vi "registers to data.vi"(6 "word order":T1, 9 "specifications":T2[](array[typedef]), 10 "registers":u16[](array[numeric]), 11 "allocation":T4) -> (3 "data table":T4)   [LabVIEW 2015, in "Modbus Module runtime.lvclass"]
uses:
  Modbus Module runtime.lvclass
  <vilib>/NI/Tag Bus/table/data table.ctl
  data mapping elements.ctl
  <vilib>/NI/Tag Bus/tag/Data Type.ctl
  <vilib>/NI/Tag Bus/table/data polymorphs/write one/write Double.vi
  <vilib>/NI/Tag Bus/table/data polymorphs/write one/write Single.vi
  <vilib>/NI/Tag Bus/table/data polymorphs/write one/write I64.vi
  <vilib>/NI/Tag Bus/table/data polymorphs/write one/write U64.vi
  <vilib>/NI/Tag Bus/table/data polymorphs/write one/write I32.vi
  <vilib>/NI/Tag Bus/table/data polymorphs/write one/write U32.vi
  <vilib>/NI/Tag Bus/table/data polymorphs/write one/write I16.vi
  <vilib>/NI/Tag Bus/table/data polymorphs/write one/write U16.vi
  <vilib>/NI/Tag Bus/table/data polymorphs/write one/write I8.vi
  <vilib>/NI/Tag Bus/table/data polymorphs/write one/write U8.vi
  <vilib>/NI/Tag Bus/table/data polymorphs/write one/write String.vi
  <vilib>/NI/Tag Bus/table/data polymorphs/write one/write Boolean.vi
  <vilib>/NI/Tag Bus/table/data table.lvlib
  <vilib>/NI/Tag Bus/tag/tag descriptor.lvclass
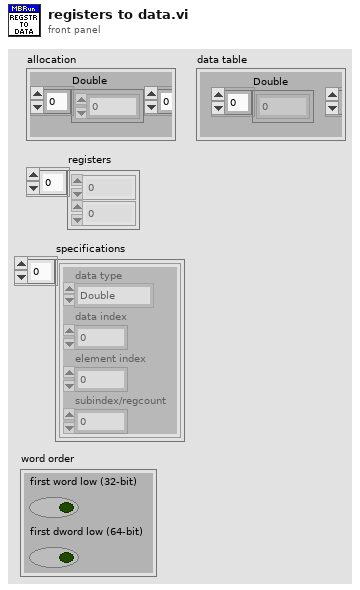
[diagram p1: front panel]
types:
  T1 = cluster{"first word low (32-bit)":bool, "first dword low (64-bit)":bool}
  T2 = typedef "Modbus Module runtime.lvclass/data mapping elements.ctl" = cluster{"data type":T3, "data index":i32, "element index":i32, "subindex/regcount":i32}
  T3 = typedef "tag bus.lvlib/tag descriptor.lvclass/Data Type.ctl" = enum16{"Double", "Single", "I64", "I32", "I16", "I8", "U64", "U32", "U16", "U8", "Boolean", "String", "Array of Double", "Array of Single", "Array of I64", "Array of I32", "Array of I16", "Array of I8", "Array of U64", "Array of U32", "Array of U16", "Array of U8", "Array of Boolean", "Array of String"}
  T4 = typedef "tag bus.lvlib/data table.lvlib/data table.ctl" = cluster{"Double":dbl[], "Single":sgl[], "I64":i64[], "I32":i32[], "I16":i16[], "I8":i8[], "U64":u64[], "U32":u32[], "U16":u16[], "U8":u8[], "Boolean":bool[], "String":string[], "Array of Double":cluster{"DBL Array":dbl[]}[], "Array of Single":cluster{"SGL Array":sgl[]}[], "Array of I64":cluster{"I64 Array":i64[]}[], "Array of I32":cluster{"I32 Array":i32[]}[], "Array of I16":cluster{"I16 Array":i16[]}[], "Array of I8":cluster{"I8 Array":i8[]}[], "Array of U64":cluster{"U64 Array":u64[]}[], "Array of U32":cluster{"U32 Array":u32[]}[], "Array of U16":cluster{"U16 Array":u16[]}[], "Array of U8":cluster{"U8 Array":u8[]}[], "Array of Boolean":cluster{"Boolean Array":bool[]}[], "Array of String":cluster{"String Array":string[]}[]}
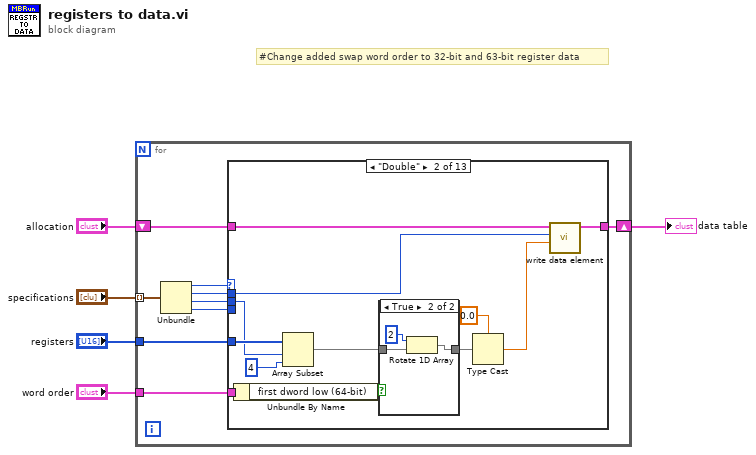
[diagram p0: block diagram]
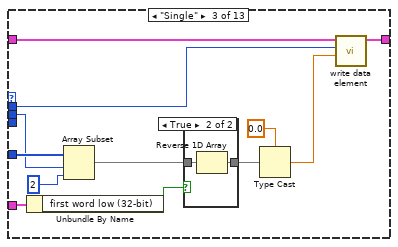
[diagram p4: hidden frame]
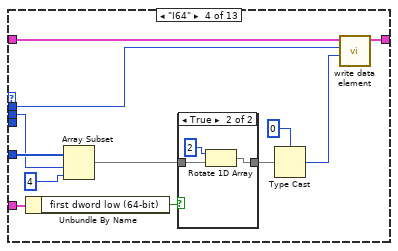
[diagram p6: hidden frame]
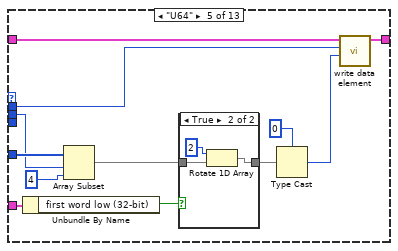
[diagram p8: hidden frame]
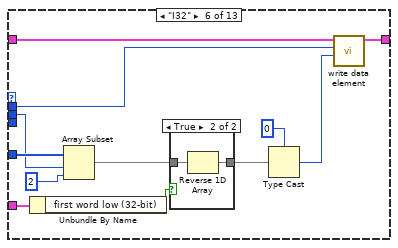
[diagram p10: hidden frame]
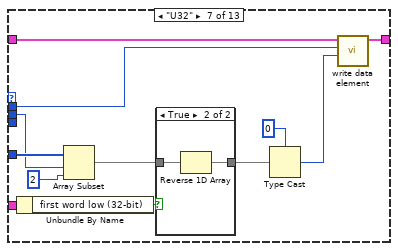
[diagram p12: hidden frame]
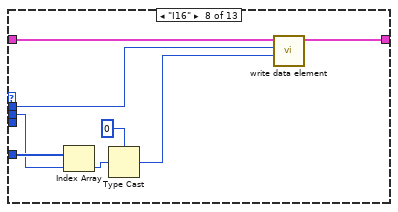
[diagram p14: hidden frame]
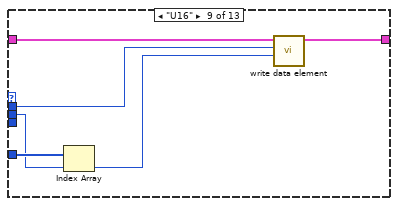
[diagram p15: hidden frame]
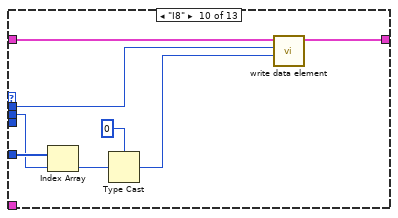
[diagram p16: hidden frame]
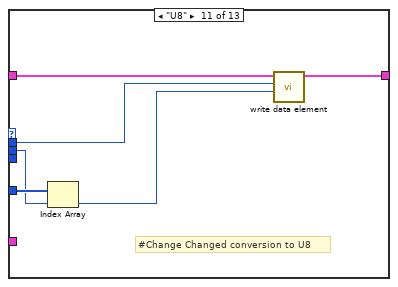
[diagram p17: hidden frame]
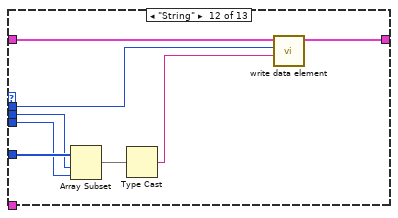
[diagram p18: hidden frame]
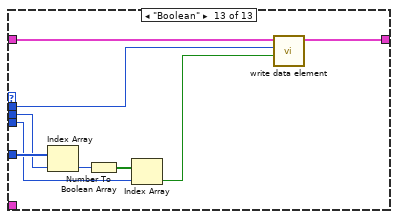
[diagram p19: hidden frame]
diagram:
  # "#Change added swap word order to 32-bit and 63-bit register data"
  n1 = for {
    shift-right: [w11] -> w4
    shift-left: "allocation" -> [w12]
    tunnel: "registers" -> [w10]
    tunnel: "specifications" -> [w14] mode=indexing
    tunnel: "word order" -> [w6]
    n2 = Unbundle(w14) -> ("data type"=w13:T3, "data index"=w9:i32, "element index"=w7:i32, "subindex/regcount"=w8:i32)
    n3 = case shown="\"Double\"" w13 {
      tunnel: w12 -> [w15 w27 w43 w58 w74 w90 w105 w116 w122 w130 w136 w144 w153]
      tunnel: [w15 w26 w42 w57 w73 w89 w104 w115 w121 w129 w135 w143 w152] -> w11
      tunnel: w7 -> [_ w23 w39 w54 w70 w86 w101 w113 w119 w127 w133 w140 w150]
      tunnel: w10 -> [_ w25 w41 w56 w72 w88 w103 w114 w120 w128 w134 w141 w151]
      tunnel: w9 -> [_ w22 w38 w53 w69 w85 w100 w112 w118 w126 w132 w142 w149]
      tunnel: w8 -> [_ _ _ _ _ _ _ _ _ _ _ w139 w145]
      tunnel: w6 -> [_ w19 w35 w48 w66 w82 w97 _ _ _ _ _ _]
      frame Default {
      }
      frame "Double" {
        n4 = Unbundle By Name(w19) -> ("first dword low (64-bit)"=w18:bool)
        n5 = Array Subset(array=w25, index=w23, length=4 ("x")) -> (w17:u16[])
        n6 = case shown="True" w18 {
          tunnel: w17 -> [w28 w31]
          tunnel: [w28 w29] -> w16
          frame False {
          }
          frame True {
            n7 = Rotate 1D Array(1:w31, 2:2 ("n")) -> (0:w29:u16[])
          }
        }
        n8 = Type Cast(type=0.0, x=w16) -> (*(type *) &x=w20:dbl)
        n9 = call-poly <vilib>:"write data element.vi"("value"=w20, "index"=w22, "data table in"=w27) -> ("data table out"=w26:T4)  [unwired: 8 in]
      }
      frame "Single" {
        n10 = Unbundle By Name(w35) -> ("first word low (32-bit)"=w34:bool)
        n11 = Array Subset(array=w41, index=w39, length=2 ("x")) -> (w33:u16[])
        n12 = case shown="True" w34 {
          tunnel: w33 -> [w44 w46]
          tunnel: [w44 w45] -> w32
          frame False {
          }
          frame True {
            n13 = Reverse 1D Array(array=w46) -> (reversed array=w45:u16[])
          }
        }
        n14 = Type Cast(type=sgl 0.0, x=w32) -> (*(type *) &x=w36:sgl)
        n15 = call-poly <vilib>:"write data element.vi"("value"=w36, "index"=w38, "data table in"=w43) -> ("data table out"=w42:T4)  [unwired: 8 in]
      }
      frame "I64" {
        n16 = Unbundle By Name(w48) -> ("first dword low (64-bit)"=w47:bool)
        n17 = Array Subset(array=w56, index=w54, length=4 ("x")) -> (w50:u16[])
        n18 = case shown="True" w47 {
          tunnel: w50 -> [w59 w62]
          tunnel: [w59 w60] -> w49
          frame False {
          }
          frame True {
            n19 = Rotate 1D Array(1:w62, 2:2 ("n")) -> (0:w60:u16[])
          }
        }
        n20 = Type Cast(type=i64 0, x=w49) -> (*(type *) &x=w51:i64)
        n21 = call-poly <vilib>:"write data element.vi"("value"=w51, "index"=w53, "data table in"=w58) -> ("data table out"=w57:T4)  [unwired: 8 in]
      }
      frame "U64" {
        n22 = Unbundle By Name(w66) -> ("first word low (32-bit)"=w65:bool)
        n23 = Array Subset(array=w72, index=w70, length=4 ("x")) -> (w64:u16[])
        n24 = case shown="True" w65 {
          tunnel: w64 -> [w75 w78]
          tunnel: [w75 w76] -> w63
          frame False {
          }
          frame True {
            n25 = Rotate 1D Array(1:w78, 2:2 ("n")) -> (0:w76:u16[])
          }
        }
        n26 = Type Cast(type=u64 0, x=w63) -> (*(type *) &x=w67:u64)
        n27 = call-poly <vilib>:"write data element.vi"("value"=w67, "index"=w69, "data table in"=w74) -> ("data table out"=w73:T4)  [unwired: 8 in]
      }
      frame "I32" {
        n28 = Unbundle By Name(w82) -> ("first word low (32-bit)"=w81:bool)
        n29 = Array Subset(array=w88, index=w86, length=2 ("x")) -> (w80:u16[])
        n30 = case shown="True" w81 {
          tunnel: w80 -> [w91 w93]
          tunnel: [w91 w92] -> w79
          frame False {
          }
          frame True {
            n31 = Reverse 1D Array(array=w93) -> (reversed array=w92:u16[])
          }
        }
        n32 = Type Cast(type=0, x=w79) -> (*(type *) &x=w83:i32)
        n33 = call-poly <vilib>:"write data element.vi"("value"=w83, "index"=w85, "data table in"=w90) -> ("data table out"=w89:T4)  [unwired: 8 in]
      }
      frame "U32" {
        n34 = Unbundle By Name(w97) -> ("first word low (32-bit)"=w96:bool)
        n35 = Array Subset(array=w103, index=w101, length=2 ("x")) -> (w95:u16[])
        n36 = case shown="True" w96 {
          tunnel: w95 -> [w106 w108]
          tunnel: [w106 w107] -> w94
          frame False {
          }
          frame True {
            n37 = Reverse 1D Array(array=w108) -> (reversed array=w107:u16[])
          }
        }
        n38 = Type Cast(type=u32 0, x=w94) -> (*(type *) &x=w98:u32)
        n39 = call-poly <vilib>:"write data element.vi"("value"=w98, "index"=w100, "data table in"=w105) -> ("data table out"=w104:T4)  [unwired: 8 in]
      }
      frame "I16" {
        n40 = Index Array(array=w114, index=w113) -> (element=w111:u16)
        n41 = Type Cast(type=i16 0, x=w111) -> (*(type *) &x=w109:i16)
        n42 = call-poly <vilib>:"write data element.vi"("value"=w109, "index"=w112, "data table in"=w116) -> ("data table out"=w115:T4)  [unwired: 8 in]
      }
      frame "U16" {
        n43 = Index Array(array=w120, index=w119) -> (element=w117:u16)
        n44 = call-poly <vilib>:"write data element.vi"("value"=w117, "index"=w118, "data table in"=w122) -> ("data table out"=w121:T4)  [unwired: 8 in]
      }
      frame "I8" {
        n45 = Index Array(array=w128, index=w127) -> (element=w125:u16)
        n46 = Type Cast(type=i8 0, x=w125) -> (*(type *) &x=w123:i8)
        n47 = call-poly <vilib>:"write data element.vi"("value"=w123, "index"=w126, "data table in"=w130) -> ("data table out"=w129:T4)  [unwired: 8 in]
      }
      frame "U8" {
        # "#Change Changed conversion to U8"
        n48 = Index Array(array=w134, index=w133) -> (element=w131:u16)
        n49 = call-poly <vilib>:"write data element.vi"("value"=w131, "index"=w132, "data table in"=w136) -> ("data table out"=w135:T4)  [unwired: 8 in]
      }
      frame "String" {
        n50 = Array Subset(array=w141, index=w140, length=w139) -> (w138:u16[])
        n51 = Type Cast(x=w138) -> (*(type *) &x=w137:string)  [unwired: 1 in]
        n52 = call-poly <vilib>:"write data element.vi"("value"=w137, "index"=w142, "data table in"=w144) -> ("data table out"=w143:T4)  [unwired: 8 in]
      }
      frame "Boolean" {
        n53 = Index Array(array=w151, index=w150) -> (element=w148:u16)
        n54 = Number To Boolean Array(number=w148) -> (Boolean array=w147:bool[])
        n55 = Index Array(array=w147, index=w145) -> (element=w146:bool)
        n56 = call-poly <vilib>:"write data element.vi"("value"=w146, "index"=w149, "data table in"=w153) -> ("data table out"=w152:T4)  [unwired: 8 in]
      }
    }
  }
  "data table" <- w4
